vi "Ensure Tool.vi"(7 "Match Type":enum16{"Full", "Suffix"}(ring), 8 "error in (no error)":errorcluster, 10 "Tool Name":string, 11 "Gantry in":refnum<class "Gantry.lvclass">) -> (0 "error out":errorcluster, 3 "Gantry out":refnum<class "Gantry.lvclass">)   [LabVIEW 2023, in "Gantry.lvclass"]
uses:
  Gantry.lvclass
  FlexWorktable/FlexWorktable.lvclass
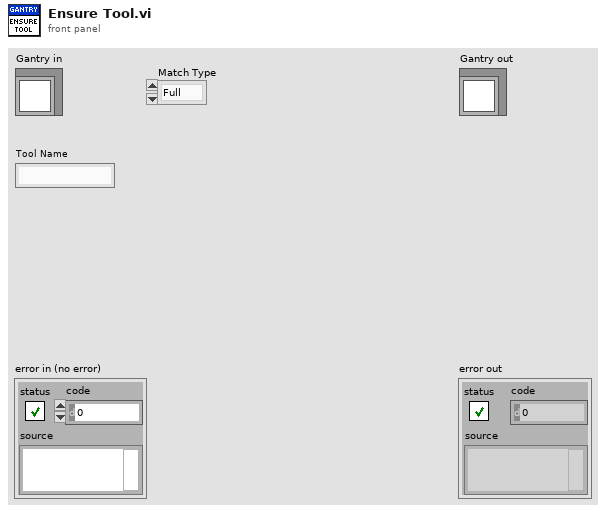
[diagram p1: front panel]
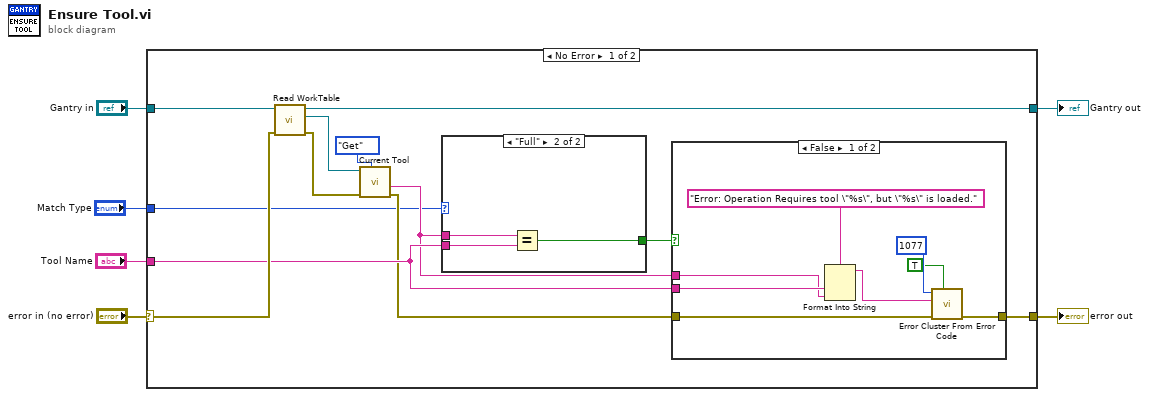
[diagram p0: block diagram]
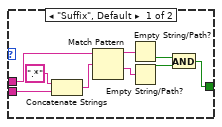
[diagram p2: hidden frame]
diagram:
  n1 = case shown="No Error" "error in (no error)" {
    selector: "error in (no error)" -> [w17 w41]
    tunnel: [w14 w41] -> w5
    tunnel: [w16 w40] -> w3
    tunnel: "Gantry in" -> [w18 w40]
    tunnel: "Tool Name" -> [w13 _]
    tunnel: "Match Type" -> [w7 _]
    frame No Error {
      n2 = call-dynamic "Read WorkTable.vi"("error in"=w17, "Gantry Class in"=w18) -> ("error out"=w10:errorcluster, "Worktable"=w12:refnum<class "FlexWorktable.lvclass">, "Gantry Class out"=w16:refnum<class "Gantry.lvclass">)  [unwired: 7 in]
      n3 = call-dynamic "Current Tool.vi"("Get/Set"=enum16{"Get", "Set"}."Get", "error in (no error)"=w10, "FlexWorktable in"=w12) -> ("error out"=w8:errorcluster, "Tool out"=w9:string)  [unwired: 5 in, 2 out]
      n4 = case shown="\"Full\"" w7 {
        tunnel: [w19 w30] -> w15
        tunnel: w13 -> [w25 w29]
        tunnel: w9 -> [w27 w28]
        frame "Suffix", Default {
          n5 = Concatenate Strings(".*" ("string"), w25) -> (w26:string)
          n6 = Match Pattern(string=w27, regular expression=w26) -> (before substring=w23:string, after substring=w22:string)  [unwired: 1 in, 2 out]
          n7 = Empty String/Path?(string/path=w23) -> (empty?=w21:bool)
          n8 = Empty String/Path?(string/path=w22) -> (empty?=w20:bool)
          n9 = And(x=w21, y=w20) -> (x .and. y?=w19:bool)
        }
        frame "Full" {
          n10 = Equal?(x=w28, y=w29) -> (x = y?=w30:bool)
        }
      }
      n11 = case shown="False" w15 {
        tunnel: w8 -> [w37 w39]
        tunnel: [w38 w39] -> w14
        tunnel: w13 -> [w33 _]
        tunnel: w9 -> [w31 _]
        frame False {
          n12 = Format Into String(format string="Error: Operation Requires tool \"%s\", but \"%s\" is loaded.", w33, w31) -> (resulting string=w32:string)  [unwired: 2 in, 1 out]
          n13 = call <vilib>:"Error Cluster From Error Code.vi"("show call chain? (False)"=TRUE, "error in (no error)"=w37, "error message (\"\")"=w32, "error code (0)"=1077) -> ("error out"=w38:errorcluster)  [unwired: 5 in]
        }
        frame True {
        }
      }
    }
    frame Error {
    }
  }
  "error out" <- w5
  "Gantry out" <- w3
